vi "MQTT_Simple_Connect_and_Publish.vi"() -> ()   [LabVIEW 2024, in "MQTT_Functions.lvlib"]
doc: "A simple client example that connects to a broker server and publishes messages to a topic.\n\n© 2015 - daq.io, LLC - Peter Adelhardt"
uses:
  MQTT_Functions.lvlib
  Controls/QoS.ctl
  Controls/Retain_Flag.ctl
  Controls/DUP_Flag.ctl
  Controls/Connection_Return_Codes.ctl
  Controls/Connect_Flags.ctl
panel:
  out "Message published":string
  in  "Stop Publishing":bool
  out "Message ID (acknowledged)":u16=10
  out "Acknowledged":bool
  in  "Message ID":u16=20
  in  "MQTT Broker":cluster{"address (IP)":string, "port":u16}={"address (IP)"="broker.hivemq.com", "port"=1883}
  in  "Message to be published":string="LabVIEW says it's "
  out "Connection Status":T1=enum."Connection refused: not authorized"
  out "error out":errorcluster
  in  "Client ID":string="LabVIEW_MQTT_Client"
  in  "error in (no error)":errorcluster
  in  "Topic":string="testtopic/LVMQTT"
  in  "Publish Meta":cluster{"QoS":T2, "Retain":T3, "DUP":T4}
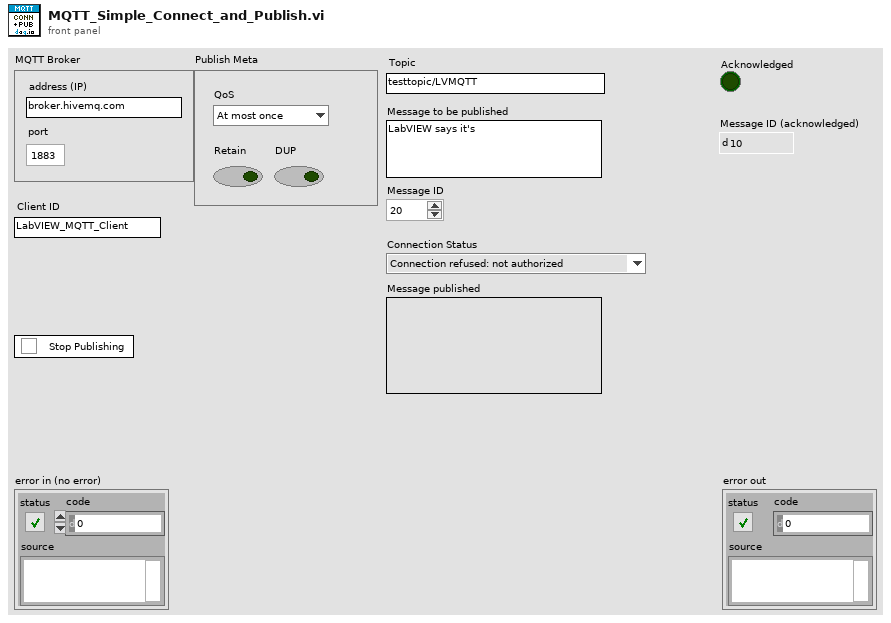
[diagram p1: front panel]
types:
  T1 = typedef "MQTT_Functions.lvlib/Connection_Return_Codes.ctl" = enum16{"Connection accepted", "Connection refused: unacceptable protocol version", "Connection refused: identifier rejected", "Connection refused: Server unavailable", "Connection refused: bad user name or password", "Connection refused: not authorized"}
  T2 = typedef "MQTT_Functions.lvlib/QoS.ctl" = enum8{"At most once", "At least once", "Exactly once", "Reserved"}
  T3 = typedef "MQTT_Functions.lvlib/Retain_Flag.ctl" = bool
  T4 = typedef "MQTT_Functions.lvlib/DUP_Flag.ctl" = bool
  T5 = typedef "MQTT_Functions.lvlib/Connect_Flags.ctl" = cluster{"user name":bool, "password":bool, "will retain":bool, "will flag":bool, "clean session":bool, "reserved":bool, "will QoS":T2}
  T6 = cluster{"QoS":T2, "DUP":T4, "Retain":T3, "Keep Alive (sec)":u16}
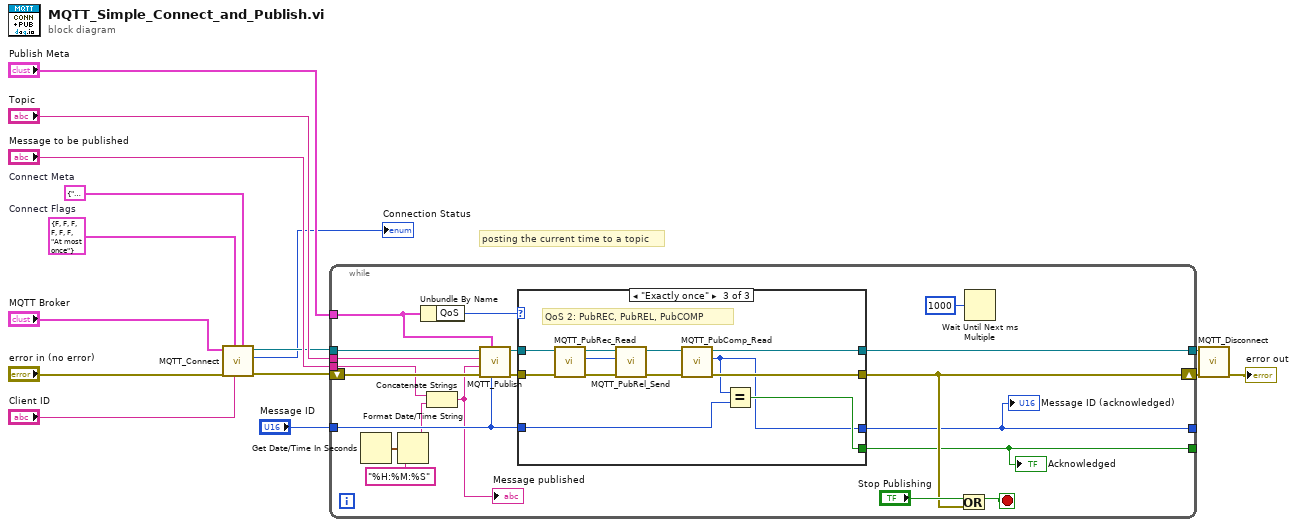
[diagram p0: block diagram]
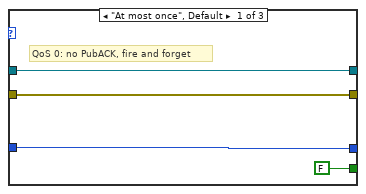
[diagram p2: hidden frame]
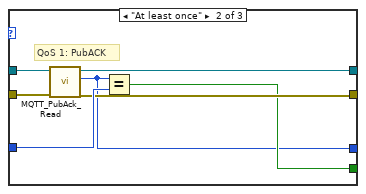
[diagram p3: hidden frame]
diagram:
  w13 = T5 {"user name"=FALSE, "password"=FALSE, "will retain"=FALSE, "will flag"=FALSE, "clean session"=FALSE, "reserved"=FALSE, "will QoS"=enum."At most once"}  # Connect Flags
  w10 = T6 {"QoS"=enum."At most once", "DUP"=FALSE, "Retain"=FALSE, "Keep Alive (sec)"=60}  # Connect Meta
  # "posting the current time to a topic"
  n1 = call "MQTT_Connect.vi"("Connect Meta"=w10, "Client ID"="Client ID", "Connect Flags"=w13, "error in (no error)"="error in (no error)", "MQTT Broker"="MQTT Broker") -> ("error out"=w1:errorcluster, "Connection Status"=→"Connection Status":T1, "connection ID out"=w3:refnum<k5>)  [unwired: 4 in]
  n2 = while {
    tunnel: "Topic" -> [w35]
    tunnel: "Message to be published" -> [w25]
    tunnel: w3 -> [w34]
    tunnel: "Publish Meta" -> [w32]
    tunnel: [w28] -> w6
    tunnel: "Message ID" -> [w27]
    tunnel: [w17] -> _
    tunnel: [w16] -> _
    shift-right: [w19] -> w7
    shift-left: w1 -> [w33]
    stop <- w20 stop-if-true
    n3 = Get Date/Time In Seconds() -> (seconds since 1Jan1904=w24:timestamp)
    n4 = Format Date/Time String(time format string (%c)="%H:%M:%S", seconds (now)=w24) -> (date/time string=w22:string)  [unwired: 1 in]
    n5 = Unbundle By Name(w32) -> ("QoS"=w31:T2)
    n6 = Concatenate Strings(w25, w22) -> (w21:string)
    "Message published" <- w21
    n7 = call "MQTT_Publish.vi"("Message ID"=w27, "Publish Meta"=w32, "error in (no error)"=w33, "Message to be published"=w21, "Topic"=w35, "connection ID"=w34) -> ("error out"=w30:errorcluster, "connection ID out"=w29:refnum<k5>)  [unwired: 4 in]
    n8 = case shown="\"Exactly once\"" w31 {
      tunnel: w30 -> [w38 w45 w57]
      tunnel: w29 -> [w39 w46 w58]
      tunnel: [w38 w43 w50] -> w19
      tunnel: [w39 w42 w51] -> w28
      tunnel: w27 -> [w36 w44 w56]
      tunnel: [FALSE w41 w52] -> w17
      tunnel: [w36 w40 w49] -> w16
      frame "At most once", Default {
        # "QoS 0: no PubACK, fire and forget"
      }
      frame "At least once" {
        # "QoS 1: PubACK"
        n9 = call "MQTT_PubAck_Read.vi"("error in (no error)"=w45, "connection ID"=w46) -> ("error out"=w43:errorcluster, "Message ID"=w40:u16, "connection ID out"=w42:refnum<k5>)  [unwired: 7 in]
        n10 = Equal?(x=w40, y=w44) -> (x = y?=w41:bool)
      }
      frame "Exactly once" {
        # "QoS 2: PubREC, PubREL, PubCOMP"
        n11 = call "MQTT_PubRec_Read.vi"("error in (no error)"=w57, "connection ID"=w58) -> ("error out"=w55:errorcluster, "Message ID"=w53:u16, "connection ID out"=w54:refnum<k5>)  [unwired: 7 in]
        n12 = call "MQTT_PubRel_Send.vi"("error in (no error)"=w55, "Message ID"=w53, "connection ID"=w54) -> ("error out"=w47:errorcluster, "connection ID out"=w48:refnum<k5>)  [unwired: 6 in, 1 out]
        n13 = call "MQTT_PubComp_Read.vi"("error in (no error)"=w47, "connection ID"=w48) -> ("error out"=w50:errorcluster, "Message ID"=w49:u16, "connection ID out"=w51:refnum<k5>)  [unwired: 7 in]
        n14 = Equal?(x=w49, y=w56) -> (x = y?=w52:bool)
      }
    }
    "Message ID (acknowledged)" <- w16
    "Acknowledged" <- w17
    n15 = Or(x="Stop Publishing", y=w19) -> (x .or. y?=w20:bool)
    n16 = Wait Until Next ms Multiple(millisecond multiple=u32 1000) -> ()  [unwired: 1 out]
  }
  n17 = call "MQTT_Disconnect.vi"("error in (no error)"=w7, "connection ID"=w6) -> ("error out"=→"error out":errorcluster)  [unwired: 9 in]
